vi "Check for New Data.vi"(5 "Set Timeout":bool, 7 "Set Pseudo PDC ID":bool, 8 "error in (no error)":errorcluster, 10 "Poll Timeout [5 ms]":i32=5, 11 "Pseudo PDC ID":i32) -> (0 "error out":errorcluster, 3 "Data Waiting":bool)   [LabVIEW 2013, in "PMU Recorder Light.lvlib" / "Statnett C37.118 DLL.lvclass"]
uses:
  Statnett C37.118 DLL.lvclass
  c37118-dll/C37118-DLL.lvlib
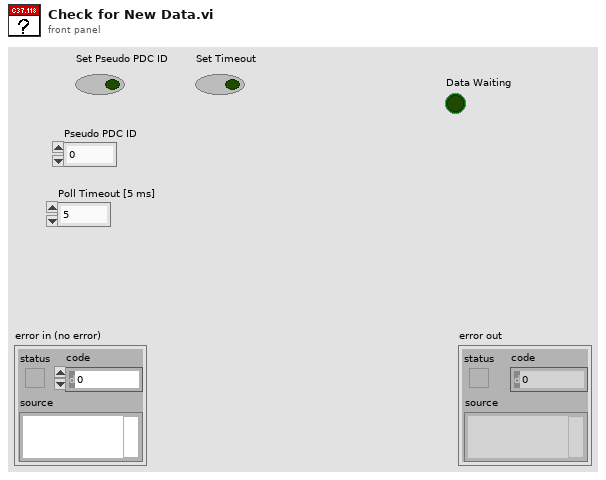
[diagram p1: front panel]
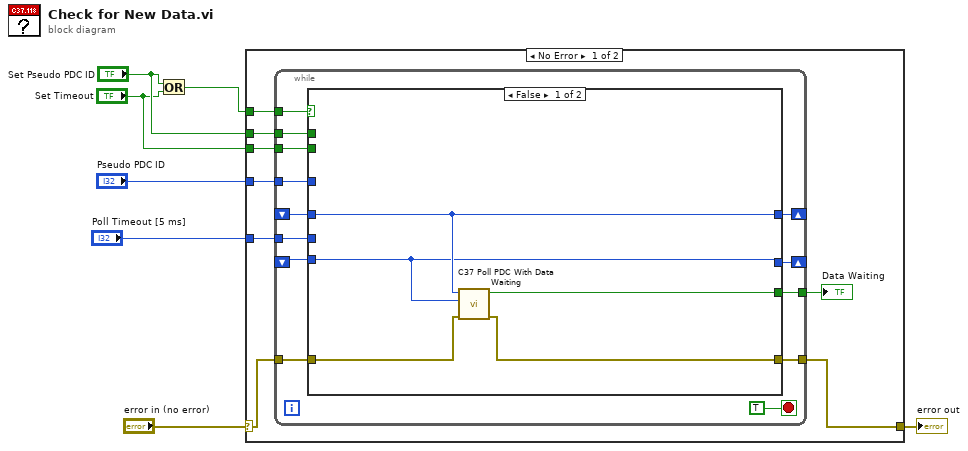
[diagram p0: block diagram]
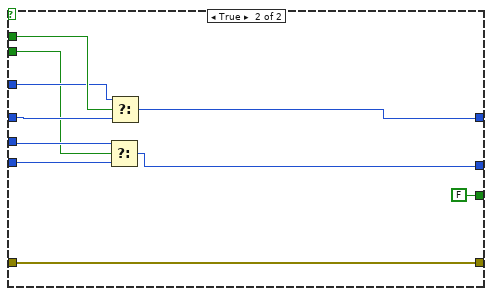
[diagram p2: hidden frame]
diagram:
  n1 = Or(x="Set Pseudo PDC ID", y="Set Timeout") -> (x .or. y?=w3:bool)
  n2 = case shown="No Error" "error in (no error)" {
    selector: "error in (no error)" -> [w15 w44]
    tunnel: [w14 w44] -> w6
    tunnel: w3 -> [w13 _]
    tunnel: "Pseudo PDC ID" -> [w12 _]
    tunnel: "Poll Timeout [5 ms]" -> [w10 _]
    tunnel: "Set Pseudo PDC ID" -> [w9 _]
    tunnel: "Set Timeout" -> [w8 _]
    frame No Error {
      n3 = while {
        tunnel: w15 -> [w28]
        tunnel: [w27] -> w14
        tunnel: w13 -> [w26]
        tunnel: w12 -> [w25]
        shift-right: [w22] -> _
        shift-left: _ -> [w23]
        tunnel: [w21] -> w11
        shift-right: [w17] -> _
        shift-left: _ -> [w16]
        tunnel: w10 -> [w20]
        tunnel: w9 -> [w19]
        tunnel: w8 -> [w18]
        stop <- TRUE stop-if-true
        n4 = case shown="False" w26 {
          tunnel: w28 -> [w30 w43]
          tunnel: [w31 w43] -> w27
          tunnel: w25 -> [_ w39]
          tunnel: w23 -> [w33 w40]
          tunnel: [w33 w38] -> w22
          tunnel: [w32 FALSE ("Data?")] -> w21
          tunnel: w20 -> [_ w37]
          tunnel: w19 -> [_ w41]
          tunnel: w18 -> [_ w36]
          tunnel: [w29 w35] -> w17
          tunnel: w16 -> [w29 w34]
          frame False {
            n5 = call "C37 Poll PDC With Data Waiting.vi"("error in (no error)"=w30, "Poll Timeout [5 ms]"=w29, "Pseudo PDC ID"=w33) -> ("error out"=w31:errorcluster, "Data?"=w32:bool)  [unwired: 7 in]
          }
          frame True {
            n6 = Select(t=w37, s=w36, f=w34) -> (s? t:f=w35:i32)
            n7 = Select(t=w39, s=w41, f=w40) -> (s? t:f=w38:i32)
          }
        }
      }
      "Data Waiting" <- w11
    }
    frame Error {
    }
  }
  "error out" <- w6
